vi "get sequence's actions.vi"(8 "error in (no error)":errorcluster, 10 "sequence name":string, 11 "Simple Sequencer TBM configuration in":refnum<class "Simple Sequencer TBM configuration.lvclass">) -> (0 "error out":errorcluster, 2 "action configs":refnum<class "action configuration.lvclass">[](array[class]), 3 "Simple Sequencer TBM configuration out":refnum<class "Simple Sequencer TBM configuration.lvclass">)   [LabVIEW 2014, in "Simple Sequencer TBM configuration.lvclass"]
doc: "Returns a list of action configurations for the specified sequence."
uses:
  Simple Sequencer TBM configuration.lvclass
  sequencer parent classes/action configuration parent/action configuration.lvclass
  Simple Sequencer TBM configuration.lvclass/Simple Sequencer TBM configuration.ctl
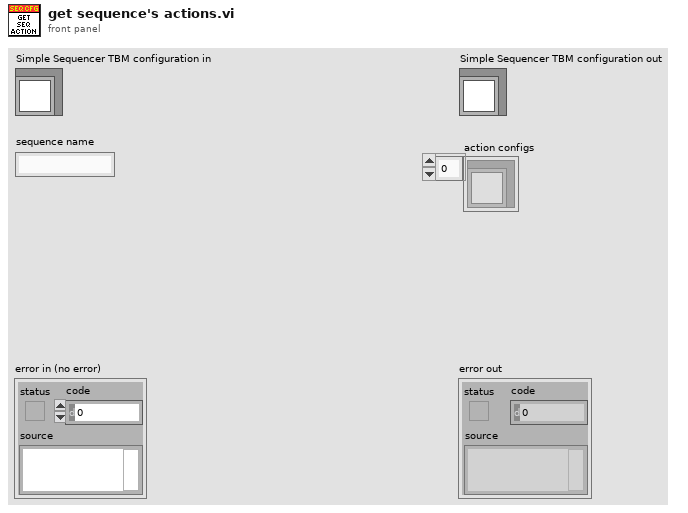
[diagram p1: front panel]
types:
  T1 = typedef "Simple Sequencer TBM configuration.lvclass/sequence definition.ctl" = cluster{"sequence name":string, "action configs":refnum<class "action configuration.lvclass">[]}
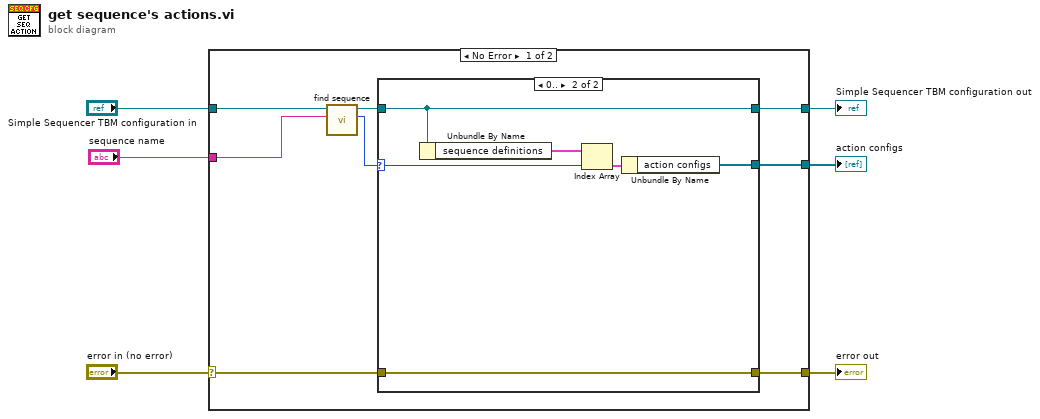
[diagram p0: block diagram]
diagram:
  n1 = case shown="No Error" "error in (no error)" {
    selector: "error in (no error)" -> [w10 w24]
    tunnel: [w9 w24] -> w5
    tunnel: [w8 w23] -> w3
    tunnel: "Simple Sequencer TBM configuration in" -> [w14 w23]
    tunnel: "sequence name" -> [w13 _]
    tunnel: [w7 _] -> w1
    frame No Error {
      n2 = call "find sequence.vi"("sequence name"=w13, "Simple Sequencer TBM configuration in"=w14) -> ("index"=w11:i32, "Simple Sequencer TBM configuration out"=w12:refnum<class "Simple Sequencer TBM configuration.lvclass">)  [unwired: 8 in]
      n3 = case shown="0.." w11 {
        selector: w11 -> [_ w20]
        tunnel: w12 -> [w15 w19]
        tunnel: w10 -> [w16 w21]
        tunnel: [w16 w21] -> w9
        tunnel: [w15 w19] -> w8
        tunnel: [_ w17] -> w7
        frame ..-1 {
          # "#todo throw error not found"
        }
        frame 0.. {
          n4 = Unbundle By Name(w19) -> ("sequence definitions"=w22:T1[])
          n5 = Index Array(array=w22, index=w20) -> (element=w18:T1)
          n6 = Unbundle By Name(w18) -> ("action configs"=w17:refnum<class "action configuration.lvclass">[])
        }
      }
    }
    frame Error {
    }
  }
  "error out" <- w5
  "Simple Sequencer TBM configuration out" <- w3
  "action configs" <- w1
